vi "rotate_lines(SubVI).vi"(6 "End X2 (m)":sgl, 7 "End Y2 (m)":sgl, 9 "centre Y1 (m)":sgl, 10 "centre X1 (m)":sgl, 11 "rotation in degrees":dbl) -> (2 "Rot End Y":dbl, 3 "Rot End X":dbl)   [LabVIEW 2014]
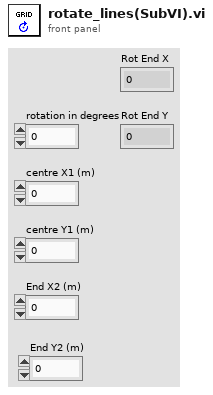
[diagram p1: front panel]
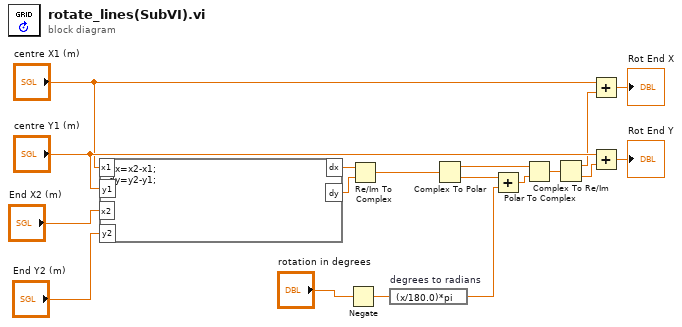
[diagram p0: block diagram]
diagram:
  n1 = formula code="dx=x2-x1;\ndy=y2-y1;"("x1"="centre X1 (m)", "x2"="End X2 (m)", "y1"="centre Y1 (m)", "y2"="End Y2 (m)") -> ("dx"=w5:dbl, "dy"=w6:dbl)
  n2 = Negate(x="rotation in degrees") -> (-x=w1:dbl)
  n3 = Re/Im To Complex(1:w6, 2:w5) -> (0:w4:cdb)
  n4 = expression code="(x/180.0)*pi" "degrees to radians"(w1) -> (w17:dbl)
  n5 = Complex To Polar(r * e^(i*theta)=w4) -> (r=w7:dbl, theta=w9:dbl)
  n6 = Add(x=w9, y=w17) -> (x+y=w8:dbl)
  n7 = Polar To Complex(1:w8, 2:w7) -> (0:w10:cdb)
  n8 = Complex To Re/Im(x + iy=w10) -> (x=w11:dbl, y=w12:dbl)
  n9 = Add(x="centre X1 (m)", y=w11) -> (x+y=→"Rot End X":dbl)
  n10 = Add(x="centre Y1 (m)", y=w12) -> (x+y=→"Rot End Y":dbl)
